vi "nome_arquivo_adq.vi"(0 "caminho":path, 1 "Configuração":string, 7 "JW":string, 9 "JK":string, 11 "JG":string, 12 "JW":bool, 13 "JK":bool, 14 "JG":bool) -> (4 "resulting string":string)   [LabVIEW 2019]
doc: "VI de criação do nome do arquivo que será salvo, utilizando as velocidades do líquido e a configuração atual."
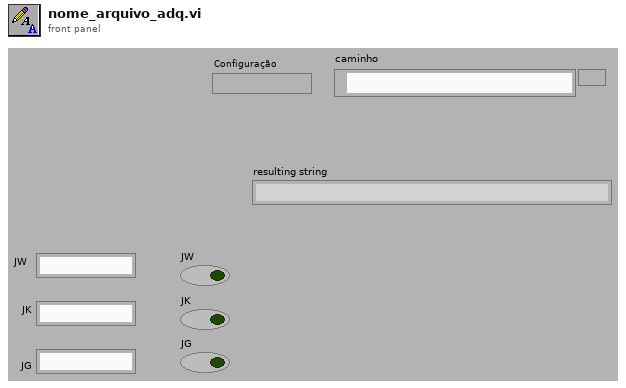
[diagram p1: front panel]
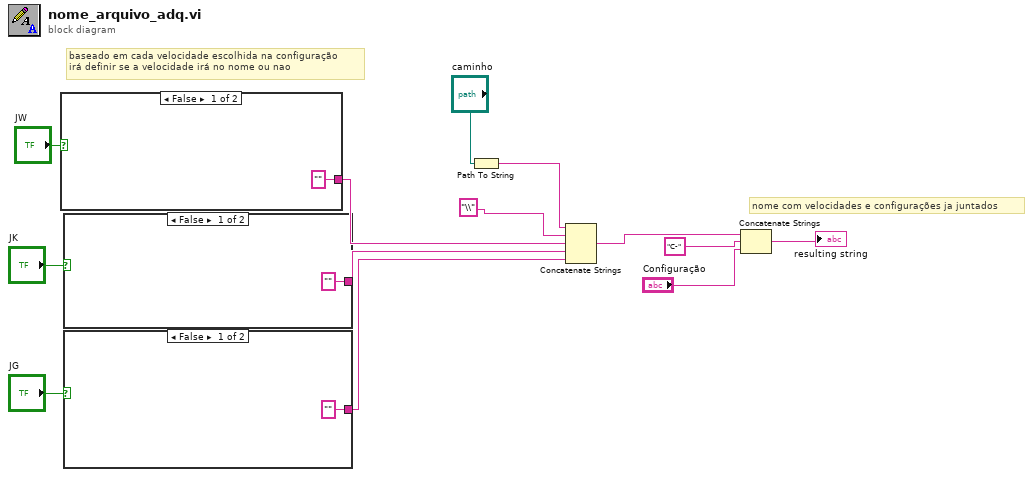
[diagram p0: block diagram]
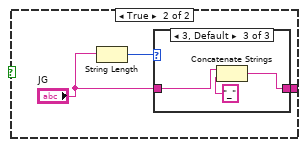
[diagram p2: hidden frame]
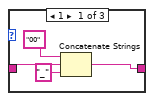
[diagram p3: hidden frame]
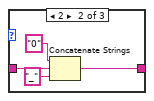
[diagram p4: hidden frame]
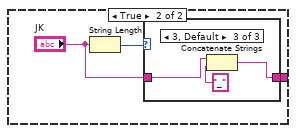
[diagram p5: hidden frame]
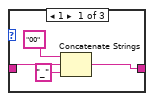
[diagram p6: hidden frame]
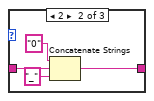
[diagram p7: hidden frame]
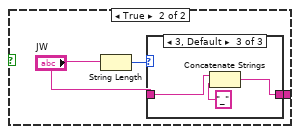
[diagram p8: hidden frame]
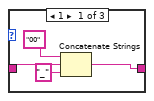
[diagram p9: hidden frame]
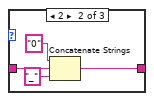
[diagram p10: hidden frame]
diagram:
  # "nome com velocidades e configurações ja juntados"
  # "baseado em cada velocidade escolhida na configuração\nirá definir se a velocidade irá no nome ou nao"
  n1 = case shown="False" "JW" {
    tunnel: ["" w15] -> w12
    frame False {
    }
    frame True {
      n2 = String Length(string="JW") -> (length=w17:i32)
      n3 = case shown="3, Default" w17 {
        tunnel: "JW" -> [w20 w24 w28]
        tunnel: [w21 w23 w26] -> w15
        frame 1 {
          n4 = Concatenate Strings("00" ("string"), w20, "_" ("string")) -> (w21:string)
        }
        frame 2 {
          n5 = Concatenate Strings("0" ("string"), w24, "_" ("string")) -> (w23:string)
        }
        frame 3, Default {
          n6 = Concatenate Strings(w28, "_" ("string")) -> (w26:string)
        }
      }
    }
  }
  n7 = case shown="False" "JK" {
    tunnel: ["" w30] -> w11
    frame False {
    }
    frame True {
      n8 = String Length(string="JK") -> (length=w32:i32)
      n9 = case shown="3, Default" w32 {
        tunnel: "JK" -> [w35 w39 w43]
        tunnel: [w36 w38 w41] -> w30
        frame 1 {
          n10 = Concatenate Strings("00" ("string"), w35, "_" ("string")) -> (w36:string)
        }
        frame 2 {
          n11 = Concatenate Strings("0" ("string"), w39, "_" ("string")) -> (w38:string)
        }
        frame 3, Default {
          n12 = Concatenate Strings(w43, "_" ("string")) -> (w41:string)
        }
      }
    }
  }
  n13 = case shown="False" "JG" {
    tunnel: ["" w47] -> w10
    frame False {
    }
    frame True {
      n14 = String Length(string="JG") -> (length=w46:i32)
      n15 = case shown="3, Default" w46 {
        tunnel: "JG" -> [w50 w54 w58]
        tunnel: [w51 w53 w56] -> w47
        frame 1 {
          n16 = Concatenate Strings("00" ("string"), w50, "_" ("string")) -> (w51:string)
        }
        frame 2 {
          n17 = Concatenate Strings("0" ("string"), w54, "_" ("string")) -> (w53:string)
        }
        frame 3, Default {
          n18 = Concatenate Strings(w58, "_" ("string")) -> (w56:string)
        }
      }
    }
  }
  n19 = Path To String(path="caminho") -> (string=w1:string)
  n20 = Concatenate Strings(w1, "\\", w12, w11, w10) -> (w9:string)
  n21 = Concatenate Strings(w9, "C-" ("input 2"), "Configuração") -> (→"resulting string":string)
